vi "ICS425 Read Write.vi"(8 "Error In":errorcluster, 10 "Cmd":string, 11 "VISA (Input)":refnum<visa-resource-name>) -> (0 "Error Out":errorcluster, 2 "read buffer":string, 3 "VISA Refnum (Output)":refnum<visa-resource-name>)   [LabVIEW 2020]
panel:
  out "Serial Settings:Number of Bytes at Serial Port":u32
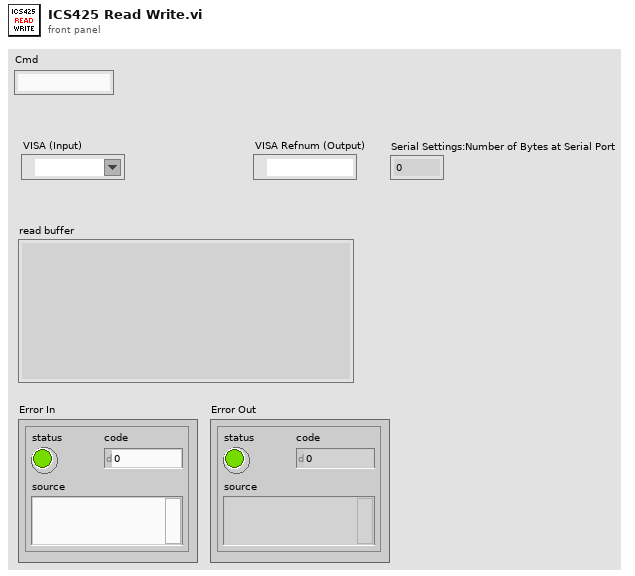
[diagram p1: front panel]
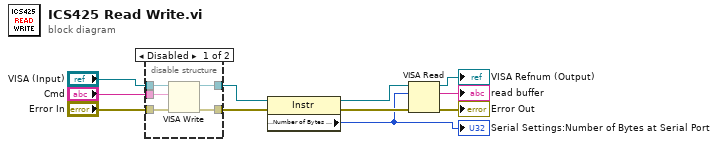
[diagram p0: block diagram]
diagram:
  n1 = disable-structure shown="Disabled" {
    disable-tunnel: "VISA (Input)" -> [w16 w18]
    disable-tunnel: [w15 w18] -> w9
    disable-tunnel: [w14 w17] -> w8
    disable-tunnel: "Error In" -> [w13 w17]
    disable-tunnel: "Cmd" -> [w12 _]
    frame Disabled {
      n2 = VISA Write(VISA resource name=w16, write buffer=w12, error in (no error)=w13) -> (VISA resource name out=w15:refnum<visa-resource-name>, error out=w14:errorcluster)  [unwired: 1 out]
    }
    frame Enabled {
    }
  }
  n3 = property class="Instr"(reference=w9, error in=w8) -> (reference out=w6:refnum<visa-resource-name>, error out=w7:errorcluster, "Serial Settings:Number of Bytes at Serial Port"=w1:u32)
  "Serial Settings:Number of Bytes at Serial Port" <- w1
  n4 = VISA Read(VISA resource name=w6, byte count=w1, error in (no error)=w7) -> (VISA resource name out=→"VISA Refnum (Output)":refnum<visa-resource-name>, read buffer=→"read buffer":string, error out=→"Error Out":errorcluster)  [unwired: 1 out]
